vi "Close.vi"(8 "error in (no error)":errorcluster, 11 "DeviceNET in":refnum<class "DeviceNET.lvclass">) -> (0 "error out":errorcluster, 3 "DeviceNET out":refnum<class "DeviceNET.lvclass">)   [LabVIEW 2016, in "DeviceNET.lvclass"]
uses:
  DeviceNET.lvclass
  DeviceNET.lvclass/DeviceNET.ctl
  Protocol Class/Protocol.lvclass
  <vilib>/DeviceNet/DeviceNetLIB.lvlib
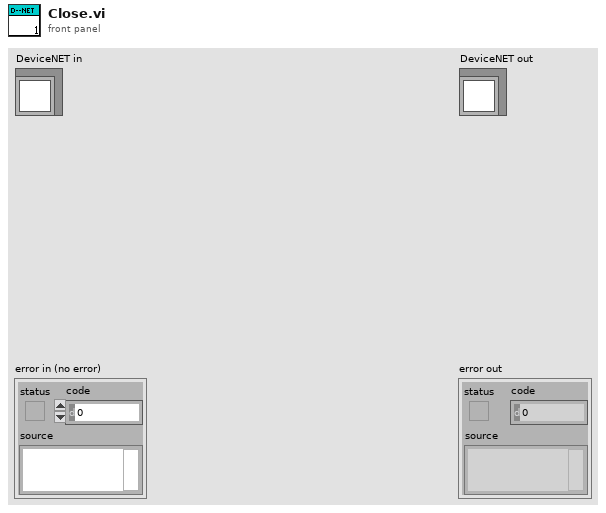
[diagram p1: front panel]
types:
  T1 = typedef "DeviceNetLIB.lvlib/xobjhandle.ctl" = u32
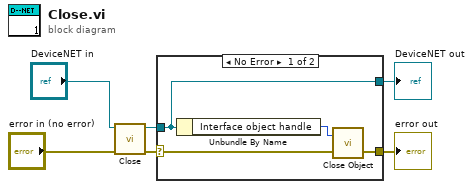
[diagram p0: block diagram]
diagram:
  n1 = call-parent "Close.vi"("error in (no error)"="error in (no error)", "Protocol in"="DeviceNET in") -> ("error out"=w4:errorcluster, "Protocol out"=w1:refnum<class "DeviceNET.lvclass">)  [unwired: 8 in]
  n2 = case shown="No Error" w4 {
    selector: w4 -> [w10 w11]
    tunnel: w1 -> [w8 w12]
    tunnel: [w8 w12] -> w2
    tunnel: [w9 w11] -> w3
    frame No Error {
      n3 = Unbundle By Name(w8) -> ("Interface object handle"=w7:T1)
      n4 = call <vilib>:"Close Object.vi"("error in (no error)"=w10, "object handle in"=w7) -> ("error out"=w9:errorcluster)  [unwired: 1 in]
    }
    frame Error {
    }
  }
  "error out" <- w3
  "DeviceNET out" <- w2
